vi "Then.vi"(8 "error in (no error)":errorcluster, 9 "Scope":variant, 10 "Callback":refnum<vi>, 11 "State in":refnum<class "State.lvclass">) -> (0 "error out":errorcluster)   [LabVIEW 2017, in "Promise Future.lvlib" / "State.lvclass"]
uses:
  State.lvclass
  State.lvclass/State.ctl
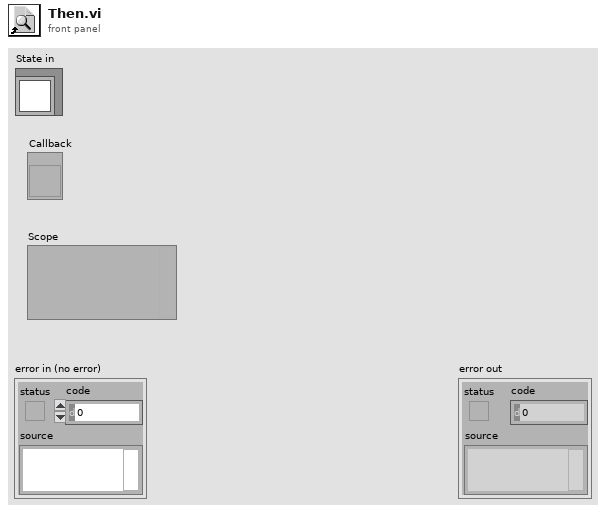
[diagram p1: front panel]
types:
  T1 = typedef "Semaphore RefNum" = refnum<k1>
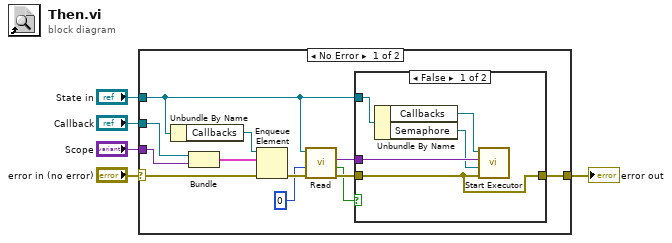
[diagram p0: block diagram]
diagram:
  n1 = case shown="No Error" "error in (no error)" {
    selector: "error in (no error)" -> [w15 w24]
    tunnel: [w14 w24] -> w4
    tunnel: "Callback" -> [w17 _]
    tunnel: "Scope" -> [w16 _]
    tunnel: "State in" -> [w7 _]
    frame No Error {
      n2 = Unbundle By Name(w7) -> ("Callbacks"=w13:refnum<queue>)
      n3 = Bundle("Callback"=w17, "Scope"=w16) -> (w6:cluster{"Callback":refnum<vi>, "Scope":variant})  [unwired: 1 in]
      n4 = Enqueue Element(queue=w13, element=w6, error in (no error)=w15) -> (error out=w12:errorcluster)  [unwired: 1 in, 2 out]
      n5 = call "Read.vi"("error in (no error)"=w12, "timeout in ms (-1)"=0, "State in"=w7) -> ("error out"=w11:errorcluster, "timed out?"=w8:bool, "Value"=w9:variant)  [unwired: 6 in]
      n6 = case shown="False" w8 {
        tunnel: w11 -> [w18 w23]
        tunnel: [w18 w23] -> w14
        tunnel: w7 -> [w21 _]
        tunnel: w9 -> [w22 _]
        frame False {
          n7 = Unbundle By Name(w21) -> ("Callbacks"=w20:refnum<queue>, "Semaphore"=w19:T1)
          n8 = call "Start Executor.vi"("error in (no error)"=w18, "semaphore"=w19, "Value"=w22, "Callbacks"=w20) -> ()  [unwired: 8 in]
        }
        frame True {
        }
      }
    }
    frame Error {
    }
  }
  "error out" <- w4
